vi "Conversion Current.vi"(8 "error in (no error)":errorcluster, 10 "Input":dbl, 11 "Top Level in":refnum<class "Top Level.lvclass">) -> (0 "error out":errorcluster, 2 "Output":dbl, 3 "Top Level out":refnum<class "Top Level.lvclass">)   [LabVIEW 2021, in "Top Level.lvlib" / "Top Level.lvclass"]
uses:
  Top Level.lvclass
  Top Level.lvclass/Top Level.ctl
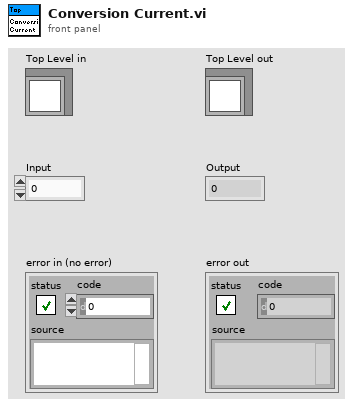
[diagram p1: front panel]
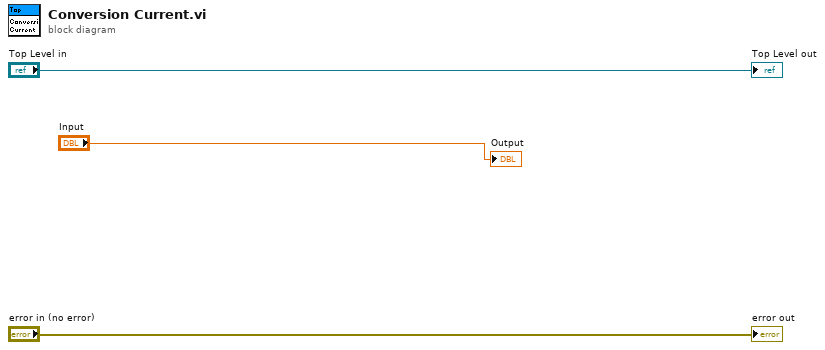
[diagram p0: block diagram]
diagram:
  "error out" <- "error in (no error)"
  "Top Level out" <- "Top Level in"
  "Output" <- "Input"
